vi "GitHub OAuth Test.vi"() -> ()   [LabVIEW 2020]
uses:
  OauthClient/OAuthClient.lvclass
  Oauth2/Oauth2.lvclass/Oauth2.ctl
  Oauth2.Github/Oauth2.GitHub.lvclass
  C:/Data/1_Projects/CIGH_Oauth2/source/Oauth2/Oauth2.lvclass
  Oauth2/Oauth2.lvclass
  <vilib>/LabVIEW Open Source Project/OpenURI/uri/URI.lvclass
  <vilib>/httpClient/LabVIEWHTTPClient.lvlib
panel:
  out "GitHub Refresh Token":string
  out "GitHub Root":string
  out "HTTP Response Headers":string
  in  "login":string
  out "error out":errorcluster
  out "GitHub Access Token":string
  in  "GitHub Client Secret":string
  in  "GitHub Client ID":string
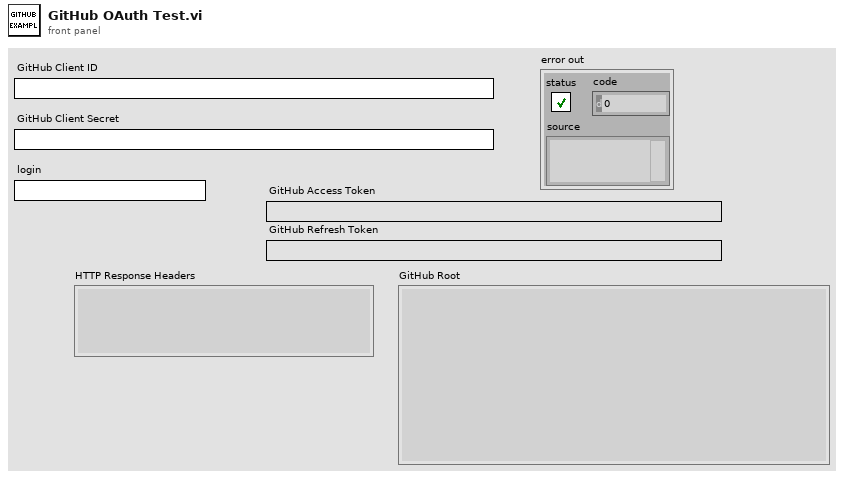
[diagram p1: front panel]
types:
  T1 = typedef "LabVIEWHTTPClient.lvlib/ClientHandle.ctl" = refnum<k1>
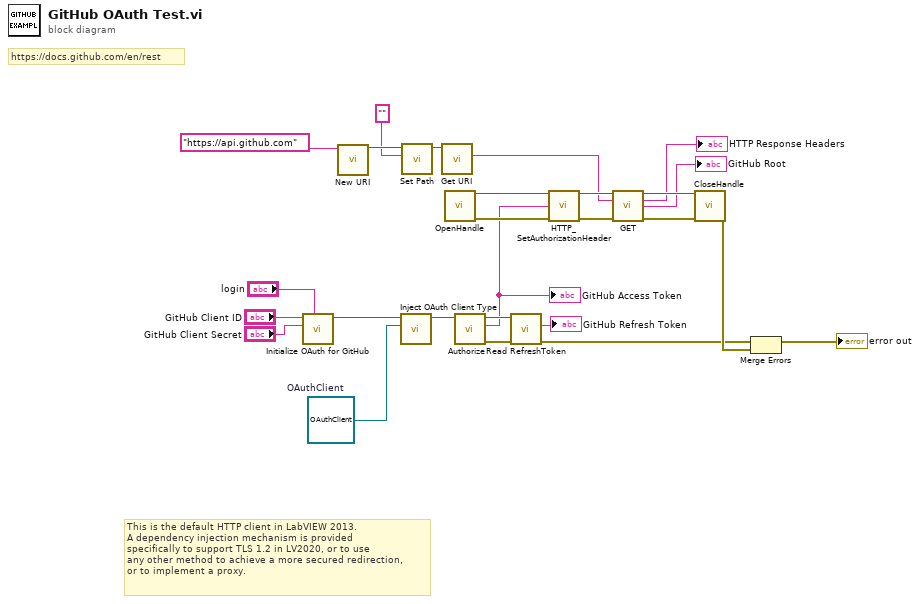
[diagram p0: block diagram]
diagram:
  w25 = refnum<class "OAuthClient.lvclass"> refnum  # OAuthClient
  # "https://docs.github.com/en/rest"
  # "This is the default HTTP client in LabVIEW 2013.\nA dependency injection mechanism is provided\nspecifically to support TLS 1.2 in LV2020, or to use\nany other method to achieve a more secured redirection, \nor to implement a proxy."
  n1 = call "Initialize OAuth for GitHub.vi"("login"="login", "Client Secret"="GitHub Client Secret", "Client ID"="GitHub Client ID") -> ("Oauth2.GitHub"=w22:refnum<class "Oauth2.GitHub.lvclass">)  [unwired: 8 in]
  n2 = call <vilib>:"New URI.vi"("URI"="https://api.github.com" ("path")) -> ("URI"=w20:refnum<class "URI.lvclass">)  [unwired: 9 in, 1 out]
  n3 = call "Inject OAuth Client Type.vi"("OAuthClient"=w25, "Oauth2 in"=w22) -> ("Oauth2"=w26:refnum<class "Oauth2.GitHub.lvclass">)  [unwired: 9 in]
  n4 = call <vilib>:"Set Path.vi"("path"="", "URI in"=w20) -> ("URI out"=w18:refnum<class "URI.lvclass">)  [unwired: 8 in, 1 out]
  n5 = call <vilib>:"Get URI.vi"("URI in"=w18) -> ("URI String"=w11:string)  [unwired: 8 in, 2 out]
  n6 = call <vilib>:"OpenHandle.vi"() -> ("client handle out"=w17:T1, "error out"=w16:errorcluster)  [unwired: 14 in]
  n7 = call "Authorize.vi"("Oauth2 in"=w26) -> ("error out"=w3:errorcluster, "Access Token"=w1:string, "Oauth2 out"=w5:refnum<class "Oauth2.GitHub.lvclass">)  [unwired: 8 in]
  "GitHub Access Token" <- w1
  n8 = call "Read RefreshToken.vi"("error in (no error)"=w3, "Oauth2 in"=w5) -> ("error out"=w2:errorcluster, "Refresh Token"=→"GitHub Refresh Token":string)  [unwired: 7 in, 1 out]
  n9 = call "HTTP_SetAuthorizationHeader.vi"("Client Handle"=w17, "Access Token"=w1, "error in (no error)"=w16) -> ("client handle dup"=w15:T1, "error out"=w14:errorcluster)  [unwired: 11 in]
  n10 = call <vilib>:"GET.vi"("client handle"=w15, "url"=w11, "error in (no error)"=w14) -> ("client handle out"=w13:T1, "headers"=→"HTTP Response Headers":string, "body"=→"GitHub Root":string, "error out"=w12:errorcluster)  [unwired: 9 in]
  n11 = call <vilib>:"CloseHandle.vi"("client handle"=w13, "error in (no error)"=w12) -> ("error out"=w8:errorcluster)  [unwired: 13 in]
  n12 = Merge Errors(w2, w8) -> (→"error out":errorcluster)
